vi "e.gate HighSpeedPort Decode Buffer Config Header Data.vi"(0 "Data in (binary)":u8[](array[numeric]), 1 "Configuration in":T1, 11 "error in (no error)":errorcluster) -> (3 "Configuration out":T1, 4 "Data out (binary)":u8[](array[numeric]), 15 "error out":errorcluster caption="error out (no error)")   [LabVIEW 2016]
doc: "This VI is used to decode all controller related information from a UDBF coded stream to the configuration cluster."
uses:
  e.gate Configuration.ctl
  e.gate Channel Data.ctl
  e.gate Data Type.ctl
  e.gate Protocol Type.ctl
  e.gate Module  Data.ctl
  e.gateHSP_DLLhandle.ctl
panel:
  out "SampleRate 2":dbl
  out "StartTime 2":dbl format="%.10f"
  out "DStartTimeToSecondFactor 2":dbl format="%.10f"
  out "StartTimeToDayFactor 2":dbl format="%.10f"
  out "ChannelCount 2":i32
  out "SampleRate":dbl
  out "StartTime":dbl format="%.10f"
  out "DStartTimeToSecondFactor":dbl format="%.10f"
  out "StartTimeToDayFactor":dbl format="%.10f"
  out "ChannelCount":i32
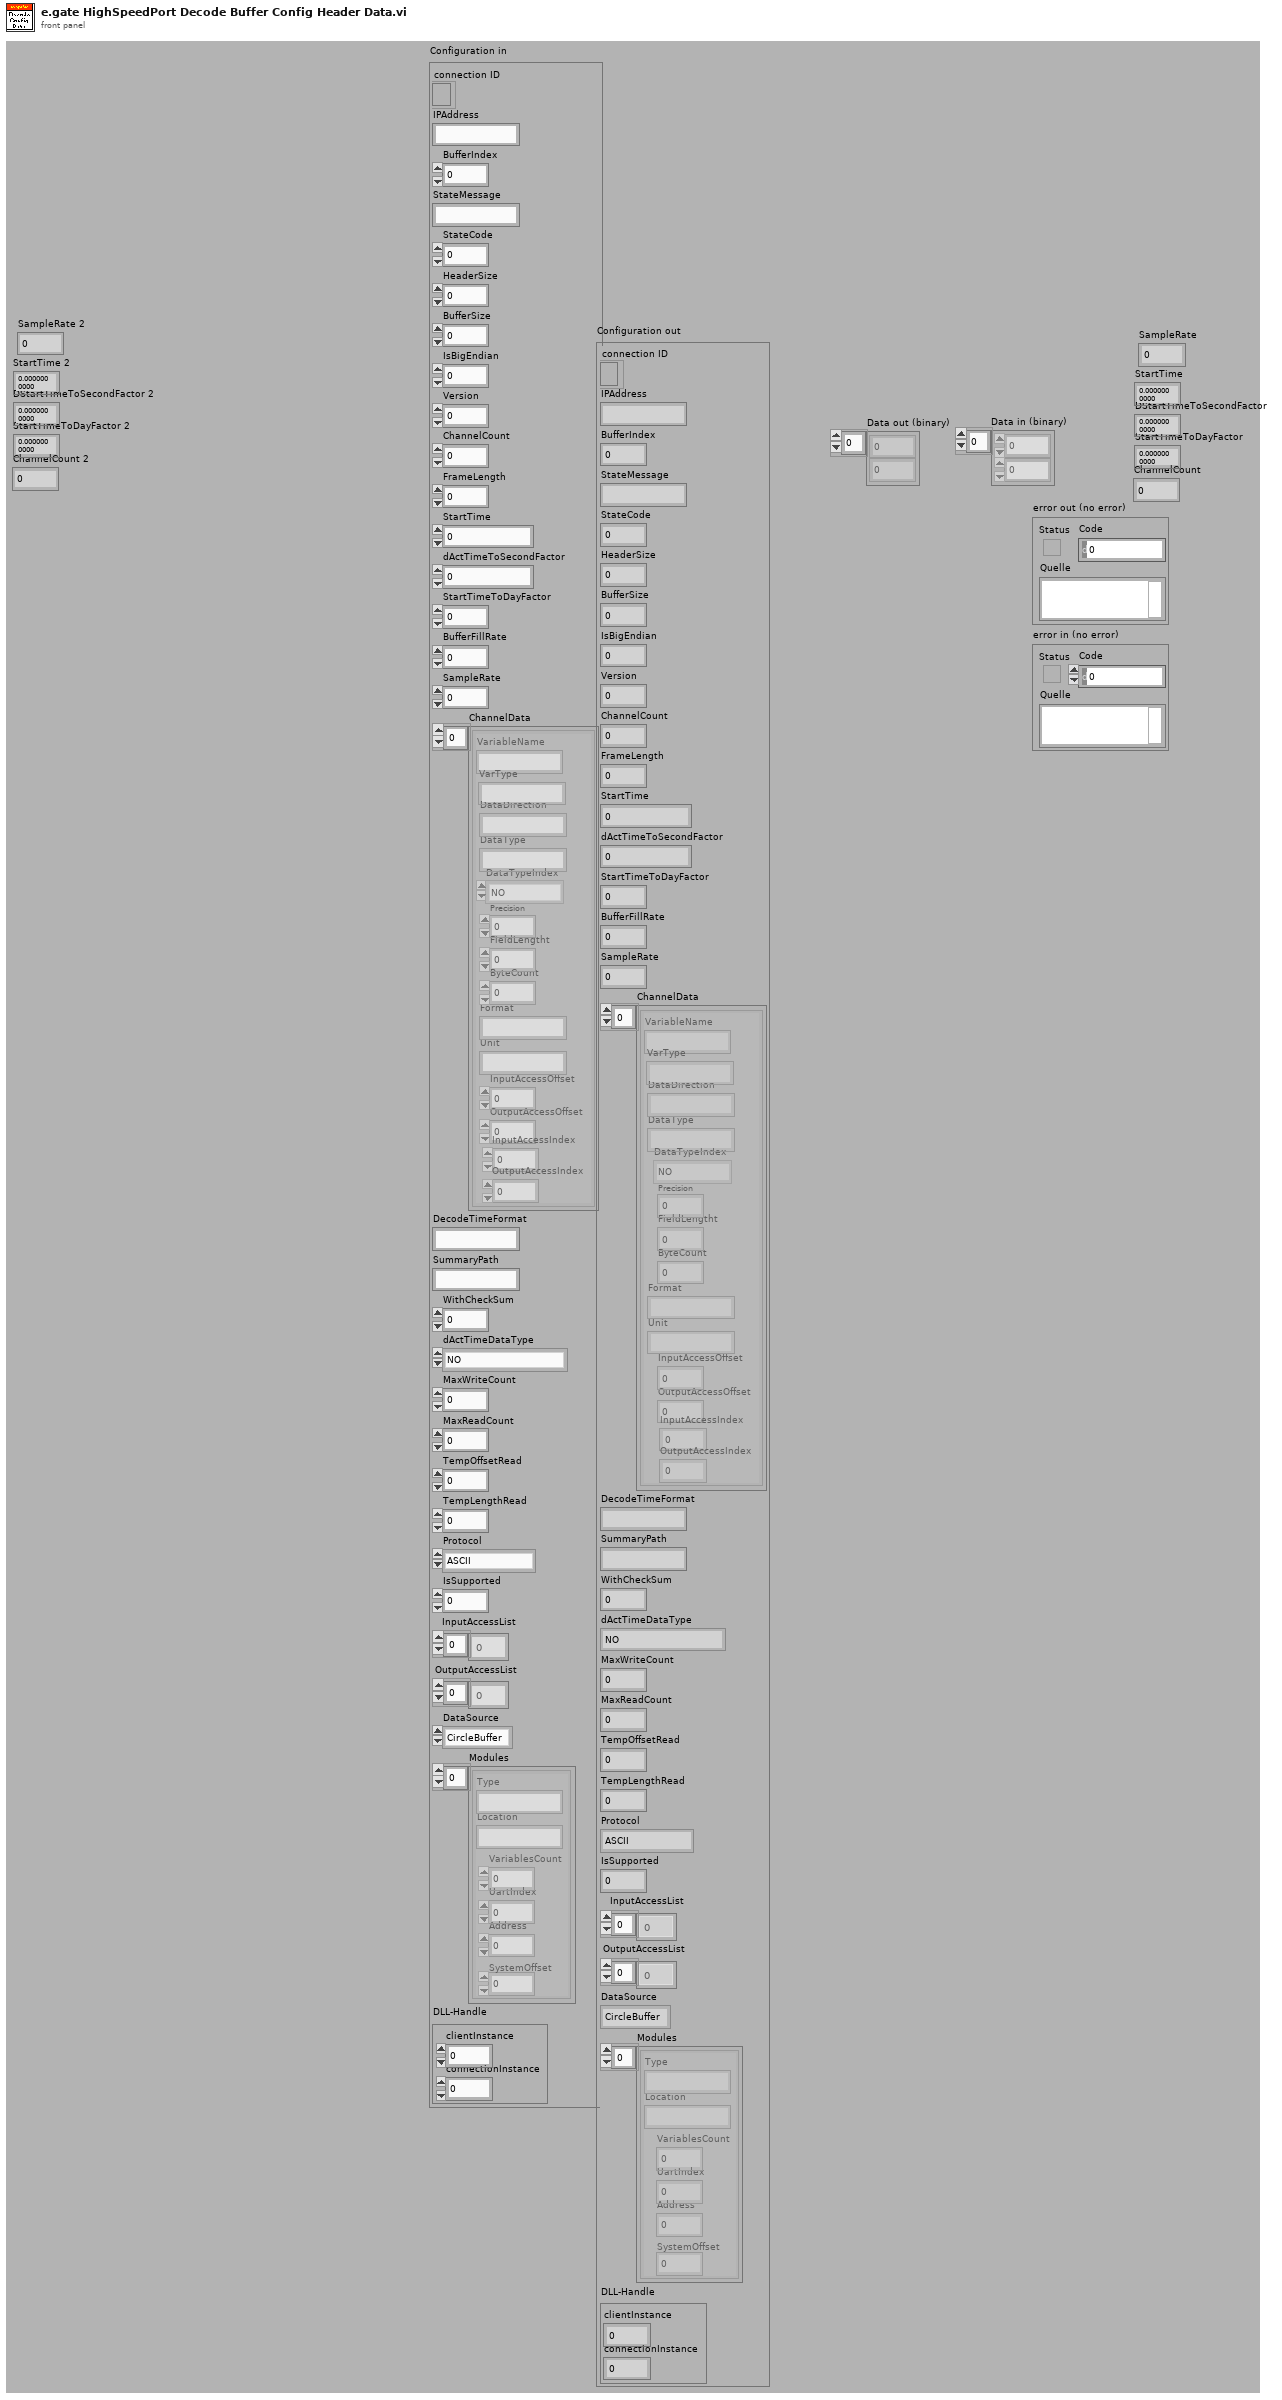
[diagram p1: front panel]
types:
  T1 = typedef "e.gate Configuration.ctl" = cluster{"connection ID":refnum<k5>, "IPAddress":string, "BufferIndex":i32, "StateMessage":string, "StateCode":i8, "HeaderSize":i32, "BufferSize":i32, "IsBigEndian":i32, "Version":i32, "ChannelCount":i32, "FrameLength":i32, "StartTime":dbl, "dActTimeToSecondFactor":dbl, "StartTimeToDayFactor":dbl, "BufferFillRate":dbl, "SampleRate":dbl, "ChannelData":T2[], "DecodeTimeFormat":string, "SummaryPath":string, "WithCheckSum":i32, "dActTimeDataType":T3, "MaxWriteCount":i32, "MaxReadCount":i32, "TempOffsetRead":i32, "TempLengthRead":i32, "Protocol":T4, "IsSupported":i32, "InputAccessList":i32[], "OutputAccessList":i32[], "DataSource":enum16{"CircleBuffer", "test.con Logger", "test.con Archive"}, "Modules":T5[], "DLL-Handle":T6}
  T2 = typedef "e.gate Channel Data.ctl" = cluster{"VariableName":string, "DataDirection":string, "DataType":string, "DataTypeIndex":T3, "Precision":i16, "FieldLengtht":i16, "ByteCount":i32, "Format":string, "Unit":string, "InputAccessOffset":i32, "OutputAccessOffset":i16, "InputAccessIndex":i16, "OutputAccessIndex":i16, "VarType":string}
  T3 = typedef "e.gate Data Type.ctl" = enum16{"NO", "BOOL", "SINT8", "USINT8", "SINT16", "USINT16", "SINT32", "USINT32", "FLOAT", "SET8", "SET16", "SET32", "DOUBLE", "SINT64", "USINT64", "SET64"}
  T4 = typedef "e.gate Protocol Type.ctl" = enum16{"ASCII", "HighspeedPort Online", "HighspeedPort Buffer", "eGateHighspeedPortDLL "}
  T5 = typedef "e.gate Module  Data.ctl" = cluster{"Type":string, "Location":string, "VariablesCount":i16, "UartIndex":i16, "Address":i16, "SystemOffset":i16}
  T6 = typedef "e.gateHSP_DLLhandle.ctl" = cluster{"clientInstance":i32, "connectionInstance":i32}
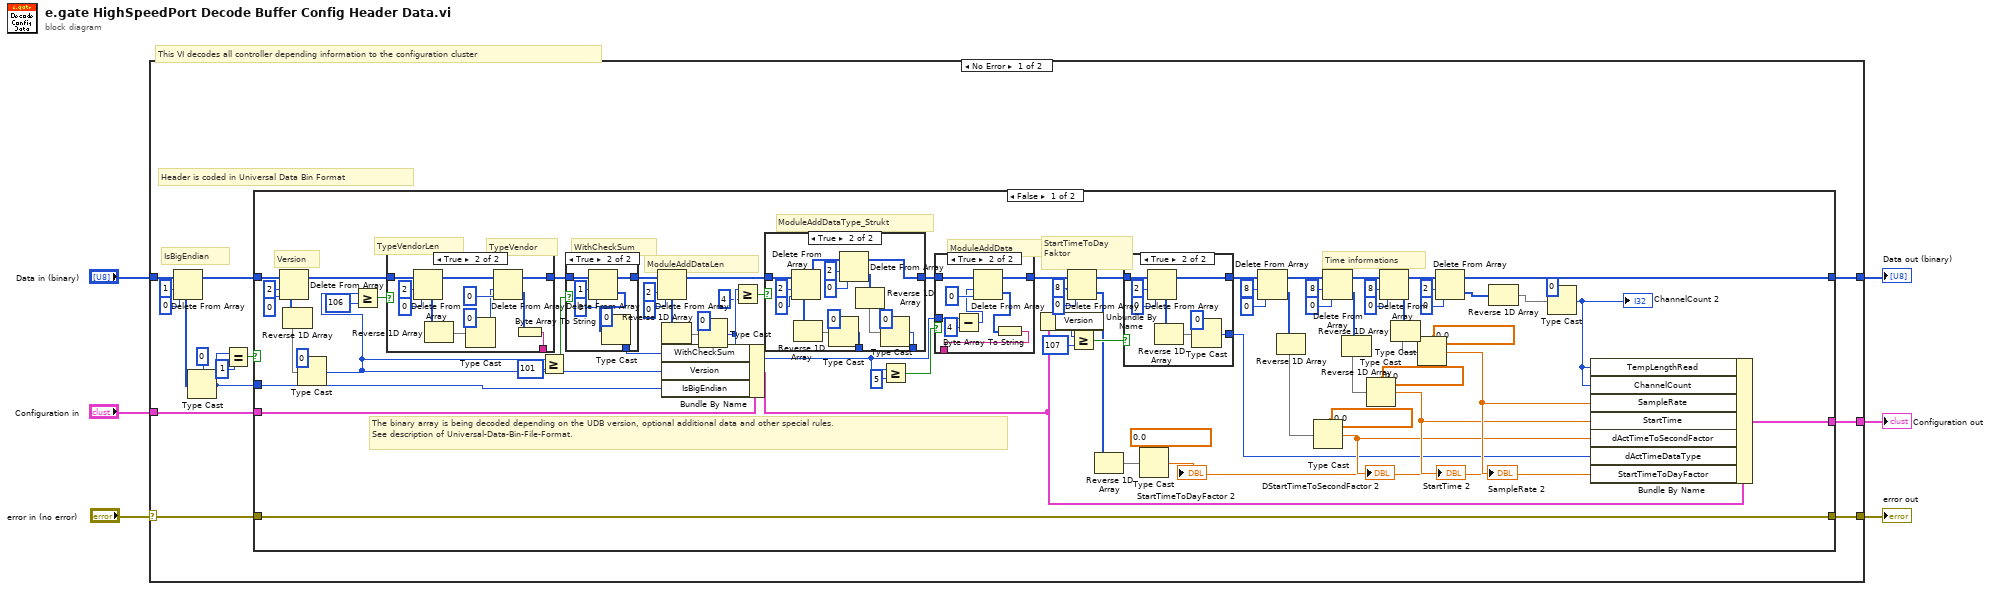
[diagram p0: block diagram]
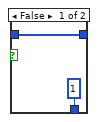
[diagram p2: hidden frame]
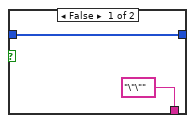
[diagram p3: hidden frame]
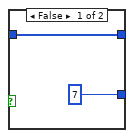
[diagram p4: hidden frame]
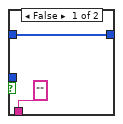
[diagram p5: hidden frame]
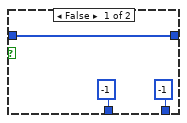
[diagram p6: hidden frame]
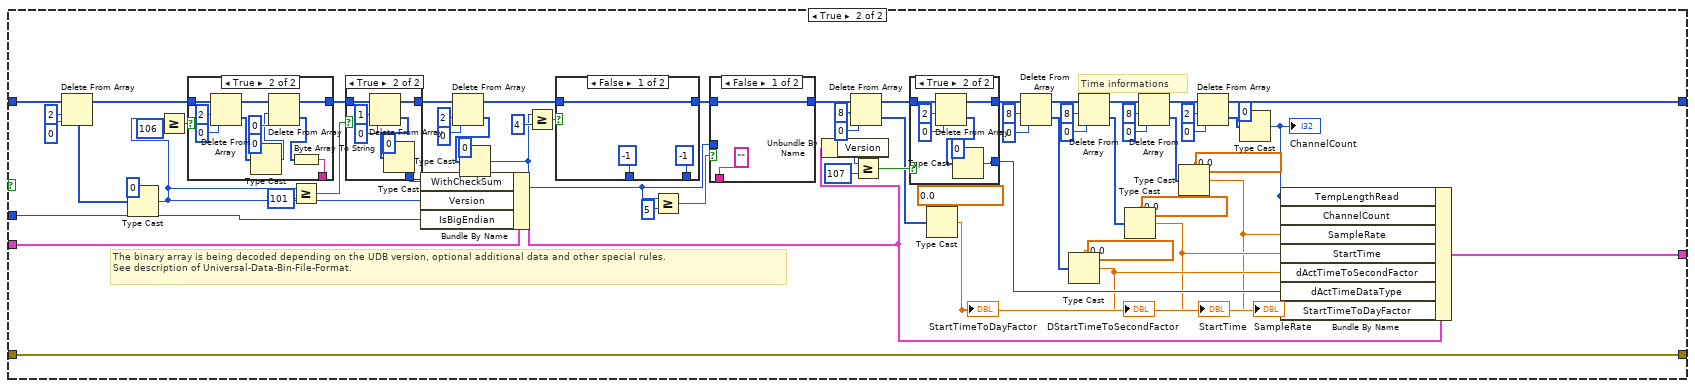
[diagram p7: hidden frame]
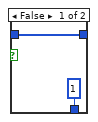
[diagram p8: hidden frame]
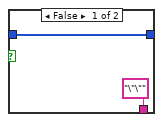
[diagram p9: hidden frame]
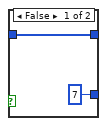
[diagram p10: hidden frame]
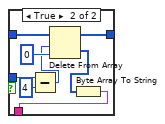
[diagram p11: hidden frame]
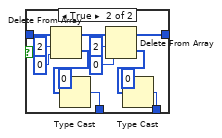
[diagram p12: hidden frame]
diagram:
  # "This VI decodes all controller depending information to the configuration cluster"
  n1 = case shown="No Error" "error in (no error)" {
    selector: "error in (no error)" -> [w8 w280]
    tunnel: "Data in (binary)" -> [w15 w279]
    tunnel: "Configuration in" -> [w14 w278]
    tunnel: [w13 w279] -> w5
    tunnel: [w7 w280] -> w4
    tunnel: [w12 w278] -> w1
    frame No Error {
      # "IsBigEndian"
      # "Header is coded in Universal Data Bin Format"
      n2 = Delete From Array(array=w15, length=1 ("Index"), index=0 ("Länge")) -> (deleted portion=w17:u8[], array with subset deleted=w19:u8[])
      n3 = Type Cast(type=i8 0, x=w17) -> (*(type *) &x=w11:i8)
      n4 = Equal?(x=w11, y=i8 1) -> (x = y?=w10:bool)
      n5 = case shown="False" w10 {
        tunnel: w19 -> [w36 w220]
        tunnel: w11 -> [w35 w170]
        tunnel: w14 -> [w39 w169]
        tunnel: [w21 w160] -> w13
        tunnel: [w30 w159] -> w12
        tunnel: w8 -> [w40 w155]
        tunnel: [w40 w155] -> w7
        frame False {
          # "StartTimeToDay\nFaktor"
          # "ModuleAddDataType_Strukt"
          # "ModuleAddData"
          # "ModuleAddDataLen"
          # "WithCheckSum"
          # "TypeVendor"
          # "TypeVendorLen"
          # "Version"
          # "Time informations"
          # "The binary array is being decoded depending on the UDB version, optional additional data and other special rules.\nSee description of Universal-Data-Bin-File-Format."
          n6 = Delete From Array(array=w36, length=2 ("Länge"), index=0 ("Index")) -> (deleted portion=w38:u8[], array with subset deleted=w41:u8[])
          n7 = Reverse 1D Array(array=w38) -> (reversed array=w37:u8[])
          n8 = Type Cast(type=i16 0, x=w37) -> (*(type *) &x=w81:i16)
          n9 = Greater Or Equal?(x=w81, y=i16 106) -> (x >= y?=w79:bool)
          n10 = case shown="True" w79 {
            tunnel: w41 -> [w104 w115]
            tunnel: [w104 w113] -> w42
            tunnel: ["\"\"" ("string") w107] -> _
            frame False {
            }
            frame True {
              n11 = Delete From Array(array=w115, length=2 ("Länge"), index=0 ("Index")) -> (deleted portion=w106:u8[], array with subset deleted=w114:u8[])
              n12 = Reverse 1D Array(array=w106) -> (reversed array=w105:u8[])
              n13 = Type Cast(type=i16 0, x=w105) -> (*(type *) &x=w108:i16)
              n14 = Delete From Array(array=w114, length=w108, index=0 ("Index")) -> (deleted portion=w112:u8[], array with subset deleted=w113:u8[])
              n15 = Byte Array To String(unsigned byte array=w112) -> (string=w107:string)
            }
          }
          n16 = Greater Or Equal?(x=w81, y=i16 101) -> (x >= y?=w82:bool)
          n17 = case shown="True" w82 {
            tunnel: w42 -> [w95 w102]
            tunnel: [w95 w101] -> w44
            tunnel: [1 w96] -> w84
            frame False {
            }
            frame True {
              n18 = Delete From Array(array=w102, length=1 ("Länge"), index=0 ("Index")) -> (deleted portion=w97:u8[], array with subset deleted=w101:u8[])
              n19 = Type Cast(type=0, x=w97) -> (*(type *) &x=w96:i32)
            }
          }
          n20 = Delete From Array(array=w44, length=2 ("Länge"), index=0 ("Index")) -> (deleted portion=w34:u8[], array with subset deleted=w50:u8[])
          n21 = Reverse 1D Array(array=w34) -> (reversed array=w33:u8[])
          n22 = Bundle By Name(cluster=w39, "WithCheckSum"=w84, "Version"=w81, "IsBigEndian"=w35) -> (w93:T1)
          n23 = Type Cast(type=0, x=w33) -> (*(type *) &x=w52:i32)
          n24 = Greater Or Equal?(x=w52, y=4) -> (x >= y?=w47:bool)
          n25 = case shown="True" w47 {
            tunnel: w50 -> [w139 w154]
            tunnel: [w139 w152] -> w51
            tunnel: [-1 w145] -> _
            tunnel: [-1 w144] -> _
            frame False {
            }
            frame True {
              n26 = Delete From Array(array=w154, length=2 ("Länge"), index=0 ("Index")) -> (deleted portion=w143:u8[], array with subset deleted=w153:u8[])
              n27 = Reverse 1D Array(array=w143) -> (reversed array=w142:u8[])
              n28 = Type Cast(type=0, x=w142) -> (*(type *) &x=w145:i32)
              n29 = Delete From Array(array=w153, length=2 ("Länge"), index=0 ("Index")) -> (deleted portion=w141:u8[], array with subset deleted=w152:u8[])
              n30 = Reverse 1D Array(array=w141) -> (reversed array=w140:u8[])
              n31 = Type Cast(type=0, x=w140) -> (*(type *) &x=w144:i32)
            }
          }
          n32 = Greater Or Equal?(x=w52, y=5) -> (x >= y?=w49:bool)
          n33 = case shown="True" w49 {
            tunnel: w51 -> [w128 w136]
            tunnel: [w128 w135] -> w53
            tunnel: w52 -> [_ w134]
            tunnel: ["" ("string") w129] -> _
            frame False {
            }
            frame True {
              n34 = Subtract(x=w134, y=4) -> (x-y=w131:i32)
              n35 = Delete From Array(array=w136, length=w131, index=0 ("Index")) -> (deleted portion=w130:u8[], array with subset deleted=w135:u8[])
              n36 = Byte Array To String(unsigned byte array=w130) -> (string=w129:string)
            }
          }
          n37 = Unbundle By Name(w93) -> ("Version"=w85:i32)
          n38 = Delete From Array(array=w53, length=8 ("Länge"), index=0 ("Index")) -> (deleted portion=w32:u8[], array with subset deleted=w73:u8[])
          n39 = Greater Or Equal?(x=w85, y=107) -> (x >= y?=w74:bool)
          n40 = Reverse 1D Array(array=w32) -> (reversed array=w31:u8[])
          n41 = case shown="True" w74 {
            tunnel: [w118 w125] -> w72
            tunnel: w73 -> [w118 w126]
            tunnel: [7 w121] -> w87
            frame False {
            }
            frame True {
              n42 = Delete From Array(array=w126, length=2 ("Länge"), index=0 ("Index")) -> (deleted portion=w120:u8[], array with subset deleted=w125:u8[])
              n43 = Reverse 1D Array(array=w120) -> (reversed array=w119:u8[])
              n44 = Type Cast(type=i16 0, x=w119) -> (*(type *) &x=w121:i16)
            }
          }
          n45 = Type Cast(type=0.0, x=w31) -> (*(type *) &x=w86:dbl)
          "StartTimeToDayFactor 2" <- w86
          n46 = Delete From Array(array=w72, length=8 ("Länge"), index=0 ("Index")) -> (deleted portion=w29:u8[], array with subset deleted=w54:u8[])
          n47 = Reverse 1D Array(array=w29) -> (reversed array=w28:u8[])
          n48 = Type Cast(type=0.0, x=w28) -> (*(type *) &x=w88:dbl)
          "DStartTimeToSecondFactor 2" <- w88
          n49 = Delete From Array(array=w54, length=8 ("Länge"), index=0 ("Index")) -> (deleted portion=w27:u8[], array with subset deleted=w55:u8[])
          n50 = Reverse 1D Array(array=w27) -> (reversed array=w26:u8[])
          n51 = Type Cast(type=0.0, x=w26) -> (*(type *) &x=w89:dbl)
          "StartTime 2" <- w89
          n52 = Delete From Array(array=w55, length=8 ("Länge"), index=0 ("Index")) -> (deleted portion=w25:u8[], array with subset deleted=w56:u8[])
          n53 = Reverse 1D Array(array=w25) -> (reversed array=w24:u8[])
          n54 = Type Cast(type=0.0, x=w24) -> (*(type *) &x=w91:dbl)
          "SampleRate 2" <- w91
          n55 = Delete From Array(array=w56, length=2 ("Länge"), index=0 ("Index")) -> (deleted portion=w23:u8[], array with subset deleted=w21:u8[])
          n56 = Reverse 1D Array(array=w23) -> (reversed array=w22:u8[])
          n57 = Type Cast(type=i16 0, x=w22) -> (*(type *) &x=w92:i16)
          "ChannelCount 2" <- w92
          n58 = Bundle By Name(cluster=w93, "TempLengthRead"=w92, "ChannelCount"=w92, "SampleRate"=w91, "StartTime"=w89, "dActTimeToSecondFactor"=w88, "dActTimeDataType"=w87, "StartTimeToDayFactor"=w86) -> (w30:T1)
        }
        frame True {
          # "Time informations"
          # "The binary array is being decoded depending on the UDB version, optional additional data and other special rules.\nSee description of Universal-Data-Bin-File-Format."
          n59 = Delete From Array(array=w220, length=2 ("Länge"), index=0 ("Index")) -> (deleted portion=w156:u8[], array with subset deleted=w219:u8[])
          n60 = Type Cast(type=i16 0, x=w156) -> (*(type *) &x=w173:i16)
          n61 = Greater Or Equal?(x=w173, y=i16 106) -> (x >= y?=w175:bool)
          n62 = case shown="True" w175 {
            tunnel: w219 -> [w231 w241]
            tunnel: [w231 w238] -> w218
            tunnel: ["\"\"" ("string") w232] -> _
            frame False {
            }
            frame True {
              n63 = Delete From Array(array=w241, length=2 ("Länge"), index=0 ("Index")) -> (deleted portion=w240:u8[], array with subset deleted=w239:u8[])
              n64 = Type Cast(type=i16 0, x=w240) -> (*(type *) &x=w233:i16)
              n65 = Delete From Array(array=w239, length=w233, index=0 ("Index")) -> (deleted portion=w237:u8[], array with subset deleted=w238:u8[])
              n66 = Byte Array To String(unsigned byte array=w237) -> (string=w232:string)
            }
          }
          n67 = Greater Or Equal?(x=w173, y=i16 101) -> (x >= y?=w172:bool)
          n68 = case shown="True" w172 {
            tunnel: w218 -> [w222 w229]
            tunnel: [w222 w228] -> w216
            tunnel: [1 w223] -> w168
            frame False {
            }
            frame True {
              n69 = Delete From Array(array=w229, length=1 ("Länge"), index=0 ("Index")) -> (deleted portion=w224:u8[], array with subset deleted=w228:u8[])
              n70 = Type Cast(type=0, x=w224) -> (*(type *) &x=w223:i32)
            }
          }
          n71 = Bundle By Name(cluster=w169, "WithCheckSum"=w168, "Version"=w173, "IsBigEndian"=w170) -> (w157:T1)
          n72 = Delete From Array(array=w216, length=2 ("Länge"), index=0 ("Index")) -> (deleted portion=w214:u8[], array with subset deleted=w209:u8[])
          n73 = Type Cast(type=0, x=w214) -> (*(type *) &x=w207:i32)
          n74 = Greater Or Equal?(x=w207, y=4) -> (x >= y?=w212:bool)
          n75 = case shown="False" w212 {
            tunnel: w209 -> [w264 w277]
            tunnel: [w264 w275] -> w208
            tunnel: [-1 w266] -> _
            tunnel: [-1 w265] -> _
            frame False {
            }
            frame True {
              n76 = Delete From Array(array=w277, length=2 ("Länge"), index=0 ("Index")) -> (deleted portion=w269:u8[], array with subset deleted=w276:u8[])
              n77 = Type Cast(type=0, x=w269) -> (*(type *) &x=w266:i32)
              n78 = Delete From Array(array=w276, length=2 ("Länge"), index=0 ("Index")) -> (deleted portion=w267:u8[], array with subset deleted=w275:u8[])
              n79 = Type Cast(type=0, x=w267) -> (*(type *) &x=w265:i32)
            }
          }
          n80 = Greater Or Equal?(x=w207, y=5) -> (x >= y?=w210:bool)
          n81 = case shown="False" w210 {
            tunnel: w208 -> [w253 w261]
            tunnel: [w253 w260] -> w206
            tunnel: w207 -> [_ w259]
            tunnel: ["" ("string") w254] -> _
            frame False {
            }
            frame True {
              n82 = Subtract(x=w259, y=4) -> (x-y=w256:i32)
              n83 = Delete From Array(array=w261, length=w256, index=0 ("Index")) -> (deleted portion=w255:u8[], array with subset deleted=w260:u8[])
              n84 = Byte Array To String(unsigned byte array=w255) -> (string=w254:string)
            }
          }
          n85 = Unbundle By Name(w157) -> ("Version"=w167:i32)
          n86 = Delete From Array(array=w206, length=8 ("Länge"), index=0 ("Index")) -> (deleted portion=w180:u8[], array with subset deleted=w185:u8[])
          n87 = Greater Or Equal?(x=w167, y=107) -> (x >= y?=w184:bool)
          n88 = case shown="True" w184 {
            tunnel: [w244 w250] -> w186
            tunnel: w185 -> [w244 w251]
            tunnel: [7 w245] -> w165
            frame False {
            }
            frame True {
              n89 = Delete From Array(array=w251, length=2 ("Länge"), index=0 ("Index")) -> (deleted portion=w246:u8[], array with subset deleted=w250:u8[])
              n90 = Type Cast(type=i16 0, x=w246) -> (*(type *) &x=w245:i16)
            }
          }
          n91 = Type Cast(type=0.0, x=w180) -> (*(type *) &x=w166:dbl)
          "StartTimeToDayFactor" <- w166
          n92 = Delete From Array(array=w186, length=8 ("Länge"), index=0 ("Index")) -> (deleted portion=w179:u8[], array with subset deleted=w205:u8[])
          n93 = Type Cast(type=0.0, x=w179) -> (*(type *) &x=w164:dbl)
          "DStartTimeToSecondFactor" <- w164
          n94 = Delete From Array(array=w205, length=8 ("Länge"), index=0 ("Index")) -> (deleted portion=w177:u8[], array with subset deleted=w204:u8[])
          n95 = Type Cast(type=0.0, x=w177) -> (*(type *) &x=w163:dbl)
          "StartTime" <- w163
          n96 = Delete From Array(array=w204, length=8 ("Länge"), index=0 ("Index")) -> (deleted portion=w176:u8[], array with subset deleted=w203:u8[])
          n97 = Type Cast(type=0.0, x=w176) -> (*(type *) &x=w161:dbl)
          "SampleRate" <- w161
          n98 = Delete From Array(array=w203, length=2 ("Länge"), index=0 ("Index")) -> (deleted portion=w201:u8[], array with subset deleted=w160:u8[])
          n99 = Type Cast(type=i16 0, x=w201) -> (*(type *) &x=w158:i16)
          "ChannelCount" <- w158
          n100 = Bundle By Name(cluster=w157, "TempLengthRead"=w158, "ChannelCount"=w158, "SampleRate"=w161, "StartTime"=w163, "dActTimeToSecondFactor"=w164, "dActTimeDataType"=w165, "StartTimeToDayFactor"=w166) -> (w159:T1)
        }
      }
    }
    frame Error {
    }
  }
  "Data out (binary)" <- w5
  "error out" <- w4
  "Configuration out" <- w1
